vi "Write statement.vi"(8 "error in (no error)":errorcluster, 10 "Statement":T1={"timestamp"=timestamp(0 s since 1904-01-01), "level"=enum."INFO", "sourceTag"="", "originVI"="", "message"=""}, 11 "LogStatementMsg in":refnum<class "LogStatementMsg.lvclass">) -> (0 "error out":errorcluster, 3 "LogStatementMsg out":refnum<class "LogStatementMsg.lvclass">)   [LabVIEW 2026, in "Lumberjack.lvlib" / "LogStatementMsg.lvclass"]
uses:
  LogStatementMsg.lvclass
  TypeDefs/Statement.ctl
  TypeDefs/Severity.ctl
  LogStatementMsg.lvclass/LogStatementMsg.ctl
  Lumberjack.lvlib
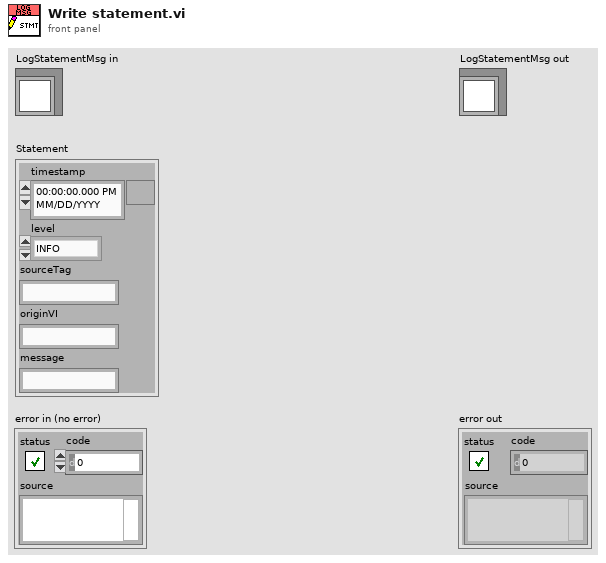
[diagram p1: front panel]
types:
  T1 = typedef "Lumberjack.lvlib/Statement.ctl" = cluster{"timestamp":timestamp, "level":T2, "sourceTag":string, "originVI":string, "message":string}
  T2 = typedef "Lumberjack.lvlib/Severity.ctl" = enum16{"OFF", "FATAL", "ERROR", "WARN", "INFO", "DEBUG", "TRACE", "ALL"}
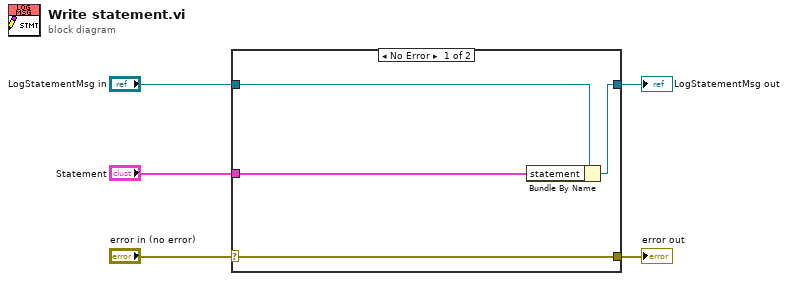
[diagram p0: block diagram]
diagram:
  n1 = case shown="No Error" "error in (no error)" {
    selector: "error in (no error)" -> [w9 w10]
    tunnel: [w9 w10] -> w4
    tunnel: [w7 w11] -> w2
    tunnel: "LogStatementMsg in" -> [w8 w11]
    tunnel: "Statement" -> [w6 _]
    frame No Error {
      n2 = Bundle By Name(cluster=w8, "statement"=w6) -> (w7:refnum<class "LogStatementMsg.lvclass">)
    }
    frame Error {
    }
  }
  "error out" <- w4
  "LogStatementMsg out" <- w2
